vi "S8300E_NETPORT_DEVICEID_WIH.vi"() -> ()   [LabVIEW 2011]
panel:
  out "PRELOG2":string
  out "PRELOG1":string
  out "log msg":string
  out "VISA resource name out":refnum<visa-resource-name>
  out "CMD-LIST":cluster{string, string, string, string}[](array[cluster])
  out "PORT3-ID":string
  out "PORT2-ID":string
  out "PORT1-ID":string
  out "BEGIN TIME":u32
  out "進行狀況":string
  # "Error Code:PORT1_ID\nError Code:PORT2_ID\nError Code:PORT3_ID"
  # "2015-6-1"
  # "S8300E Check 3 ports ID (接UART COM9)"
  # "Step1:Check UUT PORT1  DeviceID\nStep2:Check UUT PORT2  DeviceID\nStep3:Check UUT PORT3  DeviceID"
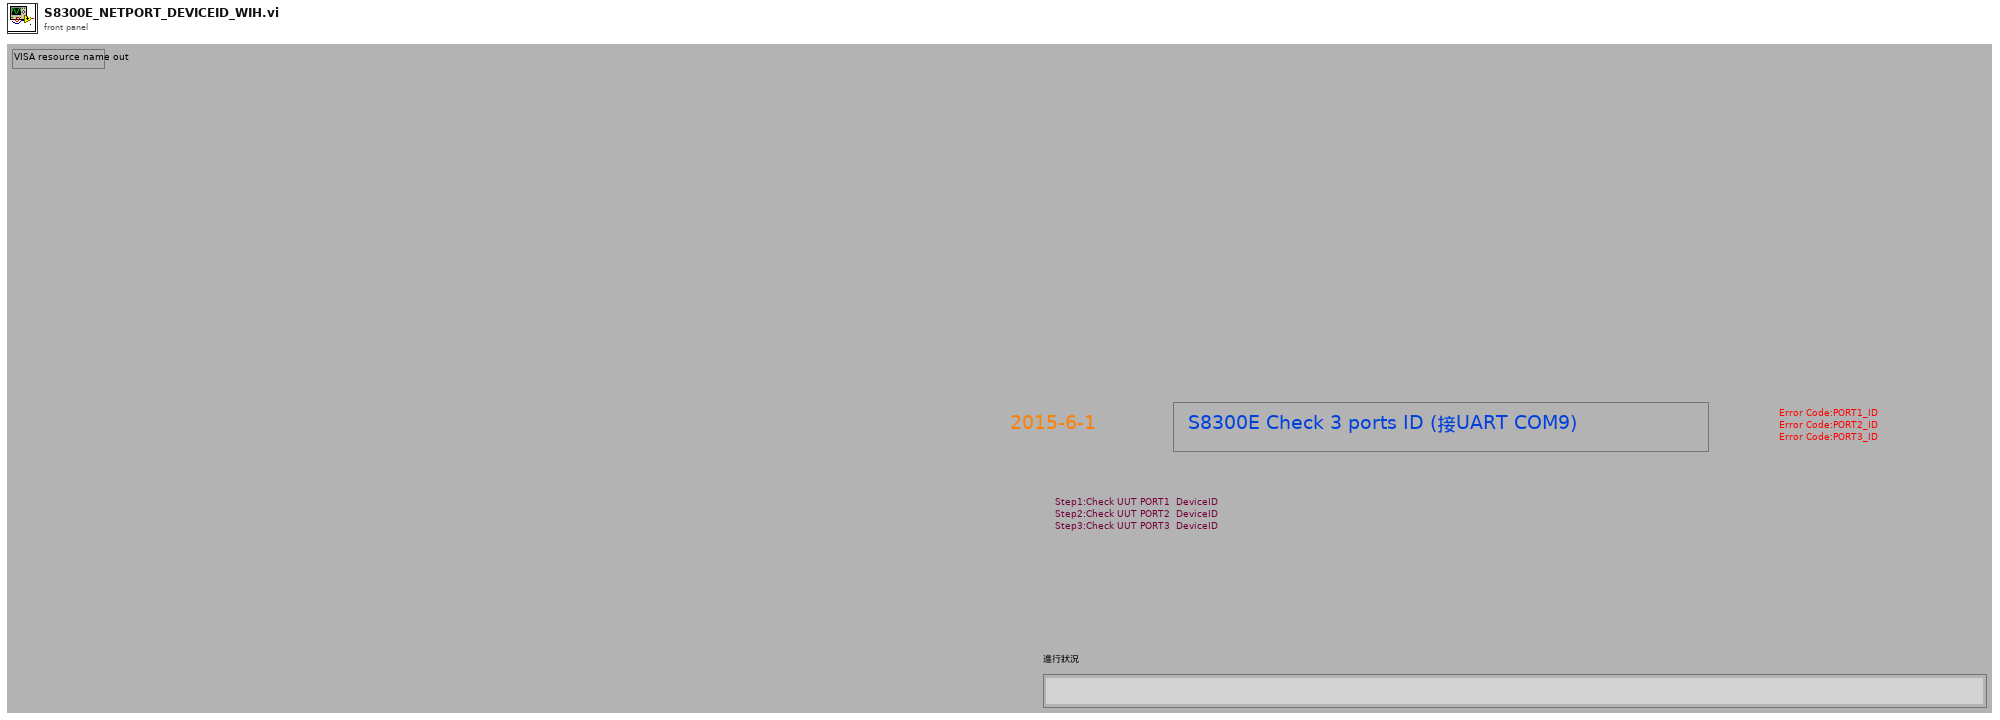
[diagram p1: front panel]
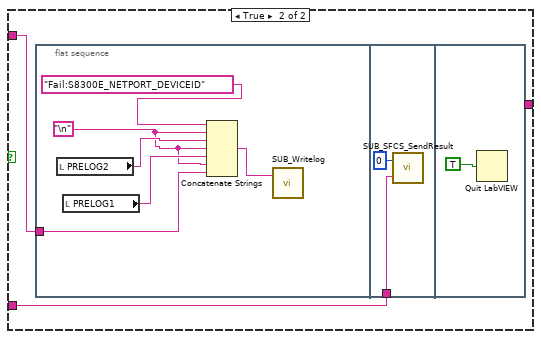
[diagram p6: hidden frame]
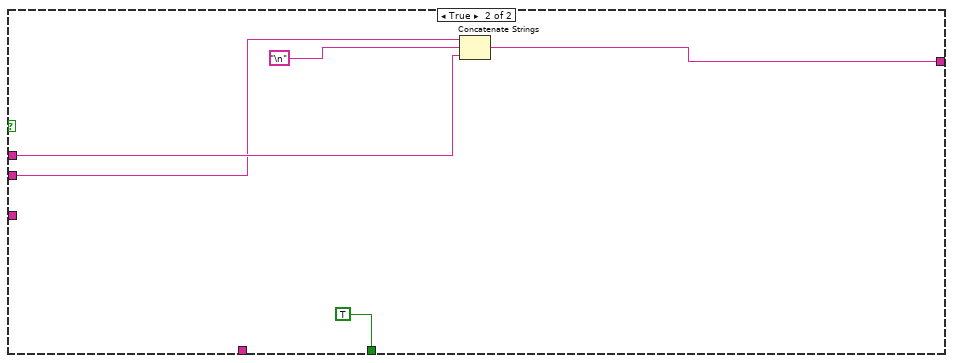
[diagram p7: hidden frame]
diagram:
  n1 = flat-sequence {
    frame #0 {
      n2 = Tick Count (ms)() -> (millisecond timer value=→"BEGIN TIME":u32)
    }
    frame #1 {
      n3 = property on="進行狀況" class="Str"("Blinking"=TRUE) -> ()  [unwired: 2 in, 2 out]
      "進行狀況" <- "進入測試準備中...." ("進行狀況")
    }
    frame #2 {
      n4 = call "SUB_SearchFile_inFolder.vi"("Search Filename in Folder"="S8300E_sfcs_misc.txt") -> ("File Existing True/Flase"=w4:bool)  [unwired: 1 in]
      n5 = case shown="False" w4 {
        frame False {
          n6 = flat-sequence {
            frame #0 {
              n7 = call "Display Message to User"() -> ()  [unwired: 10 in, 2 out]
            }
            frame #1 {
              n8 = call "SUB_Writelog.vi"("Pass/Fail"="Fail:S8300E_NETPORT_DEVICEID") -> ()  [unwired: 2 in]
            }
            frame #2 {
              n9 = Quit LabVIEW(quit? (T)=TRUE) -> ()
            }
          }
        }
        frame True {
        }
      }
    }
    frame #3 {
      n10 = call "SUB_ReadScript_File.vi"("Script FileName"="S8300E_sfcs_misc.txt" ("Search Filename in Folder")) -> ("text"=w16:string)  [unwired: 1 in, 2 out]
      n11 = call "SUB_FindSpecificString.vi"("Find this String"="UUT_PORT2_DEVICE_ID=", "String data"=w16) -> ("before \"; \" string"=→"PORT2-ID":string, "Found"=w14:bool)  [unwired: 2 in]
      n12 = call "SUB_FindSpecificString.vi"("Find this String"="UUT_PORT3_DEVICE_ID=", "String data"=w16) -> ("before \"; \" string"=→"PORT3-ID":string, "Found"=w12:bool)  [unwired: 2 in]
      n13 = call "SUB_FindSpecificString.vi"("Find this String"="UUT_PORT1_DEVICE_ID=", "String data"=w16) -> ("before \"; \" string"=→"PORT1-ID":string, "Found"=w15:bool)  [unwired: 2 in]
      n14 = And(x=w15, y=w14) -> (x .and. y?=w13:bool)
      n15 = And(x=w13, y=w12) -> (x .and. y?=w11:bool)
      n16 = case shown="False" w11 {
        frame False {
          n17 = flat-sequence {
            frame #0 {
              n18 = call "Display Message to User2"() -> ()  [unwired: 10 in, 2 out]
            }
            frame #1 {
              n19 = call "SUB_Writelog.vi"("Pass/Fail"="Fail:S8300E_NETPORT_DEVICEID") -> ()  [unwired: 2 in]
            }
            frame #2 {
              n20 = Quit LabVIEW(quit? (T)=TRUE) -> ()
            }
          }
        }
        frame True {
        }
      }
    }
    frame #4 {
      n21 = local read "PORT1-ID"() -> (w47:string)
      n22 = local read "PORT2-ID"() -> (w40:string)
      n23 = local read "PORT3-ID"() -> (w39:string)
      n24 = Concatenate Strings("PASSED=", w47) -> (w37:string)
      n25 = Concatenate Strings("./eth.sh -d  1", "\r") -> (w38:string)
      n26 = Concatenate Strings("./eth.sh -d  2", "\r") -> (w35:string)
      n27 = Concatenate Strings("PASSED=", w40) -> (w34:string)
      n28 = Concatenate Strings("./eth.sh -d  3", "\r") -> (w32:string)
      n29 = Concatenate Strings("PASSED=", w39) -> (w31:string)
      n30 = Bundle(w35, w34, "Check PORT2  DEVICE ID .....", "PORT2_ID") -> (w25:cluster{string, string, string, string})  [unwired: 1 in]
      n31 = Bundle(w32, w31, "Check PORT3  DEVICE ID .....", "PORT3_ID") -> (w24:cluster{string, string, string, string})  [unwired: 1 in]
      n32 = Bundle(w38, w37, "Check PORT1 DEVICE ID .....", "PORT1_ID") -> (w29:cluster{string, string, string, string})  [unwired: 1 in]
      n33 = Build Array(w29, w25, w24) -> (→"CMD-LIST":cluster{string, string, string, string}[])
    }
    frame #5 {
      n34 = case shown="True" TRUE {
        frame False {
        }
        frame True {
          n35 = call "SUB_COM1_CLOSE.vi"("VISA resource name"=refnum<visa-resource-name> "COM9") -> ()  [unwired: 3 in]
        }
      }
    }
    frame #6 {
      n36 = case shown="True" TRUE {
        frame False {
        }
        frame True {
          n37 = call "SUB_COM9_INIT.vi"("baud rate"=u32 115200) -> ("VISA resource name out"=w57:refnum<visa-resource-name>)  [unwired: 1 in, 1 out]
          "VISA resource name out" <- w57
          n38 = call "SUB_COM1Wrt.vi"("VISA resource name"=w57, "write buffer"="\r") -> ("duplicate VISA resource name"=w54:refnum<visa-resource-name>)  [unwired: 1 in, 1 out]
          n39 = call "SUB_ContinueCom1Read.vi"("Numeric"=3600, "duplicate VISA resource name 2"=w54) -> ()  [unwired: 1 in, 3 out]
        }
      }
    }
    frame #7 {
      n40 = local read "CMD-LIST"() -> (w62:cluster{string, string, string, string}[])
      n41 = Array Size(array=w62) -> (size(s)=w61:i32)
      n42 = for {
        N: w61 -> [_]
        shift-right: [w64] -> w59
        shift-left: "" -> [w63]
        i -> [w67]
        n43 = while {
          tunnel: w67 -> [w86]
          shift-right: [w71] -> w65
          shift-left: "" -> [w70]
          stop <- w79 stop-if-true
          n44 = local read "VISA resource name out"() -> (w73:refnum<visa-resource-name>)
          n45 = local read "CMD-LIST"() -> (w85:cluster{string, string, string, string}[])
          n46 = call "SUB_ContinueCom1Read.vi"("Numeric"=1200, "duplicate VISA resource name 2"=w73) -> ("duplicate VISA resource name"=w72:refnum<visa-resource-name>)  [unwired: 1 in, 2 out]
          n47 = Index Array(array=w85, index=w86) -> (element=w81:cluster{string, string, string, string})
          n48 = Unbundle(w81) -> (w68:string, w76:string, w78:string, w75:string)
          n49 = call "SUB_COM1Wrt.vi"("VISA resource name"=w72, "write buffer"=w68) -> ("duplicate VISA resource name"=w84:refnum<visa-resource-name>)  [unwired: 1 in, 1 out]
          n50 = Tick Count (ms)() -> (millisecond timer value=w83:u32)
          n51 = call "SUB_READ_COM1_FindString_timeout.vi"("Find this String"=w76, "Timeout Seccond"=2.0, "Begin time"=w83, "duplicate VISA resource name 2"=w84) -> ("Output String"=w77:string, "Found String"=w80:bool)  [unwired: 1 in, 1 out]
          n52 = local write "進行狀況"(w78) -> ()
          n53 = case shown="False" w80 {
            tunnel: [_ TRUE] -> w79
            tunnel: w78 -> [w96 _]
            tunnel: w77 -> [w89 w113]
            tunnel: w75 -> [w92 _]
            tunnel: [w88 w112] -> w69
            tunnel: w68 -> [_ w111]
            frame False {
              n54 = Concatenate Strings("與定義不符!" ("string"), w96) -> (w91:string)
              n55 = call "SUB_YESNO.vi"("Debug View"=w89, "Status"=w91) -> ("yes/no"=w95:enum32{"No Selection", "Yes", "No", "None"})  [unwired: 1 in]
              n56 = Equal?(x=w95, y=enum32{"No Selection", "Yes", "No", "None"}."No") -> (x = y?=w93:bool)
              n57 = Concatenate Strings(w91, "\n", w89) -> (w87:string)
              n58 = case shown="False" w93 {
                tunnel: w92 -> [_ w100]
                tunnel: [w98 _] -> w88
                tunnel: w87 -> [w98 w99]
                frame False {
                }
                frame True {
                  n59 = flat-sequence {
                    tunnel: w99 -> [w101]
                    tunnel: w100 -> [w107]
                    frame #0 {
                      w103 = "\n"
                      n60 = local read "PRELOG2"() -> (w105:string)
                      n61 = local read "PRELOG1"() -> (w104:string)
                      n62 = Concatenate Strings("Fail:S8300E_NETPORT_DEVICEID" ("Pass/Fail"), w103, w105, w103, w104, w103, w101) -> (w102:string)
                      n63 = call "SUB_Writelog.vi"("Pass/Fail"=w102) -> ()  [unwired: 2 in]
                    }
                    frame #1 {
                      n64 = call "SUB_SFCS_SendResult.vi"("ErrorCode"=w107, "PASS_Fail (1/0)"=i8 0) -> ()  [unwired: 1 out]
                    }
                    frame #2 {
                      n65 = Quit LabVIEW(quit? (T)=TRUE) -> ()
                    }
                  }
                }
              }
            }
            frame True {
              n66 = Concatenate Strings(w111, "\n", w113) -> (w112:string)
            }
          }
          n67 = Concatenate Strings(w70, w69) -> (w71:string)
          "PRELOG1" <- w71
        }
        n68 = Concatenate Strings(w63, w65) -> (w64:string)
        "PRELOG2" <- w64
      }
      "log msg" <- w59
    }
    frame #8 {
      n69 = call "SUB_COM1_CLOSE.vi"("VISA resource name"=refnum<visa-resource-name> "COM9") -> ()  [unwired: 3 in]
    }
    frame #9 {
      w118 = "***Not Good ***" ("replace string (\"\")")
      n70 = local read "log msg"() -> (w122:string)
      n71 = local read "BEGIN TIME"() -> (w127:u32)
      n72 = Tick Count (ms)() -> (millisecond timer value=w126:u32)
      n73 = call "SUB_CAL_TESTTIME.vi"("Test Item name"="S8300E_NETPORT_DEVICEID", "Stop tick time"=w126, "Start tick time"=w127) -> ("Test Time output"=w124:string)  [unwired: 2 in]
      n74 = Concatenate Strings("Pass:S8300E_NETPORT_DEVICEID", "\n", w122, w124) -> (w117:string)
      n75 = call "SUB_SEARCH_REPLACE_STR.vi"("replace string (\"\")"=w118, "search string"="FAILED", "input string"=w117) -> ("result string"=w120:string)  [unwired: 2 in]
      n76 = call "SUB_SEARCH_REPLACE_STR.vi"("replace string (\"\")"=w118, "search string"="FAIL", "input string"=w120) -> ("result string"=w116:string)  [unwired: 2 in]
      n77 = call "SUB_Writelog.vi"("Pass/Fail"=w116) -> ()  [unwired: 2 in]
    }
    frame #10 {
      n78 = Request Deallocation(TRUE ("flag")) -> ()
    }
    frame #11 {
      n79 = Quit LabVIEW(quit? (T)=TRUE ("stop? (T)")) -> ()
    }
  }
